vi "RD Digital In Read.vi"(7 "backsize":i32, 8 "error in (no error)":errorcluster caption="错误输入（无错误）", 9 "RxBuffer":u16[](array[numeric])=array[20001 elements], 10 "size":i32, 11 "handle":u64) -> (0 "error out":errorcluster caption="错误输出", 1 "RxBuffer out":u16[](array[numeric]), 2 "function return":i32, 3 "handle out":u64, 5 "backsize out":i32)   [LabVIEW 2018, in "InstrumentsPlayground.lvlib"]
doc: "CLIFFAPI int CliffDigitalInRead(FT_HANDLE handle,int size,UINT16* RxBuffer,int *backsize);\nread ditial IO In's data"
uses:
  InstrumentsPlayground.lvlib
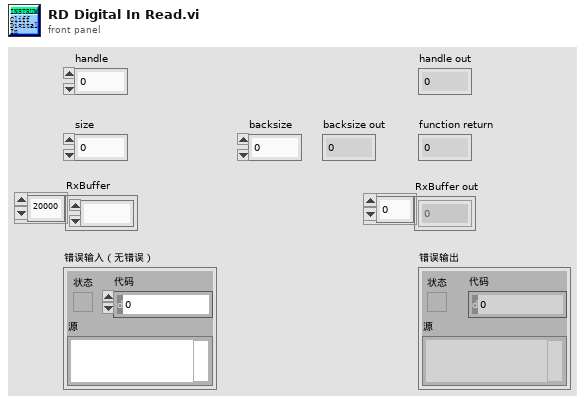
[diagram p1: front panel]
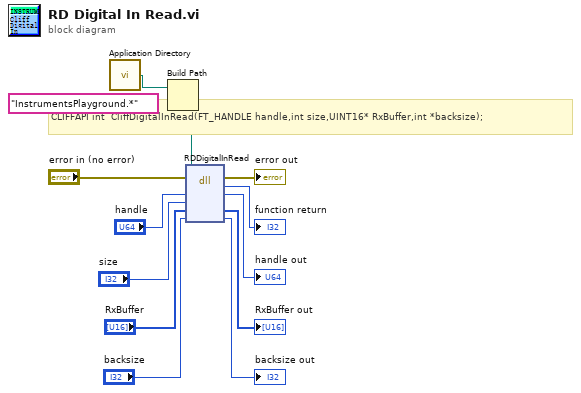
[diagram p0: block diagram]
diagram:
  # "CLIFFAPI int  CliffDigitalInRead(FT_HANDLE handle,int size,UINT16* RxBuffer,int *backsize);"
  n1 = call <vilib>:"Application Directory.vi"() -> ("Application Directory"=w2:path)
  n2 = Build Path(base path=w2, name or relative path="InstrumentsPlayground.*" ("名称或相对路径")) -> (appended path=w1:path)
  n3 = dll-call lib="E:/work/YZCourse_Xtext/Cliff/API/LabVIEW lib/InstrumentsPlayground.*" fn="RDDigitalInRead"(path in=w1, error in="error in (no error)", "handle"="handle", "size"="size", "RxBuffer"="RxBuffer", "backsize"="backsize") -> (error out=→"error out":errorcluster, "返回类型"=→"function return":i32, "handle"=→"handle out":u64, "RxBuffer"=→"RxBuffer out":u16[], "backsize"=→"backsize out":i32)  [unwired: 2 in, 1 out]
